vi "CreateOffsetFormulaINI.vi"(2 "error in (no error)":errorcluster, 3 "configuration file path":path) -> (0 "error out":errorcluster, 1 "file path":path)   [LabVIEW 2012]
uses:
  <vilib>/Utility/config.llb/Write Key (String).vi
  <vilib>/Utility/config.llb/NI_LVConfig.lvlib
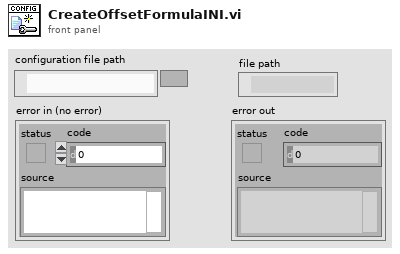
[diagram p1: front panel]
types:
  T1 = typedef "NI_LVConfig.lvlib/Config Data RefNum.ctl" = refnum<k1>
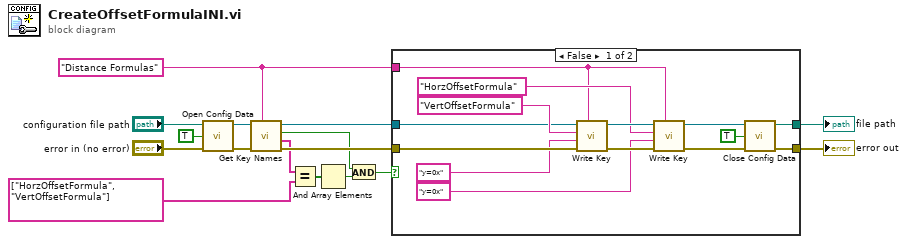
[diagram p0: block diagram]
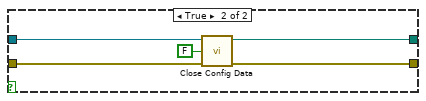
[diagram p2: hidden frame]
diagram:
  w11 = "Distance Formulas"
  n1 = call <vilib>:"Open Config Data.vi"("error in (no error)"="error in (no error)", "create file if necessary (T)"=TRUE, "configuration file path"="configuration file path") -> ("error out"=w12:errorcluster, "refnum"=w13:T1)  [unwired: 6 in, 1 out]
  n2 = call <vilib>:"Get Key Names.vi"("section"=w11, "error in (no error)"=w12, "refnum"=w13) -> ("error out"=w9:errorcluster, "key names"=w8:string[], "section exists?"=w4:bool, "refnum out"=w10:T1)  [unwired: 5 in]
  n3 = Equal?(x=w8, y=string[] ["HorzOffsetFormula", "VertOffsetFormula"]) -> (x = y?=w6:bool[])
  n4 = And Array Elements(Boolean array=w6) -> (logical AND=w5:bool)
  n5 = And(x=w4, y=w5) -> (x .and. y?=w2:bool)
  n6 = case shown="False" w2 {
    tunnel: w11 -> [w23 _]
    tunnel: w10 -> [w22 w31]
    tunnel: w9 -> [w21 w32]
    tunnel: [w20 w34] -> w1
    tunnel: [w19 w33] -> w3
    frame False {
      n7 = call-poly <vilib>:"Write Key.vi"("section"=w23, "error in (no error)"=w21, "value"="y=0x", "key"="VertOffsetFormula", "refnum"=w22) -> ("error out"=w28:errorcluster, "refnum out"=w29:T1)  [unwired: 4 in, 1 out]
      n8 = call-poly <vilib>:"Write Key.vi"("section"=w23, "error in (no error)"=w28, "value"="y=0x", "key"="HorzOffsetFormula", "refnum"=w29) -> ("error out"=w27:errorcluster, "refnum out"=w26:T1)  [unwired: 4 in, 1 out]
      n9 = call <vilib>:"Close Config Data.vi"("error in (no error)"=w27, "write file if changed (T)"=TRUE, "refnum"=w26) -> ("error out"=w19:errorcluster, "file path"=w20:path)  [unwired: 7 in]
    }
    frame True {
      n10 = call <vilib>:"Close Config Data.vi"("error in (no error)"=w32, "write file if changed (T)"=FALSE, "refnum"=w31) -> ("error out"=w33:errorcluster, "file path"=w34:path)  [unwired: 7 in]
    }
  }
  "file path" <- w1
  "error out" <- w3
